vi "Create Screen.vi"(8 "error in (no error)":errorcluster caption="错误输入（无错误）", 11 "Screen 输入":refnum<class "Screen.lvclass"> caption="DNL_LabVIEW Object in") -> (0 "error out":errorcluster caption="错误输出", 3 "Screen 输出":refnum<class "Screen.lvclass"> caption="DNL_LabVIEW Object out")   [LabVIEW 2011, in "Screen.lvclass"]
uses:
  Screen.lvclass
  Screen.lvclass/Screen.ctl
  System.Windows.Forms
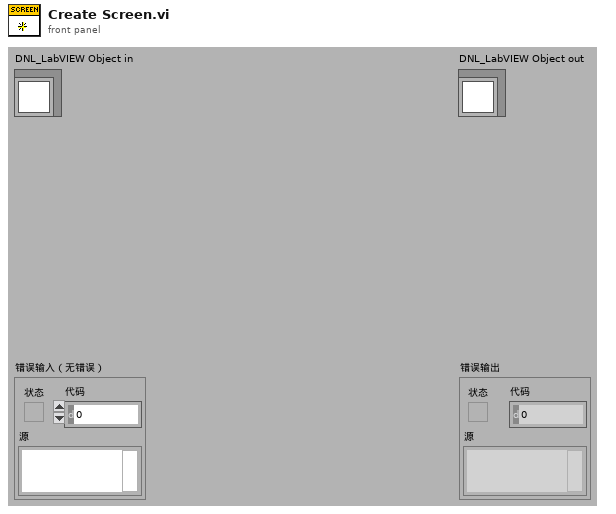
[diagram p1: front panel]
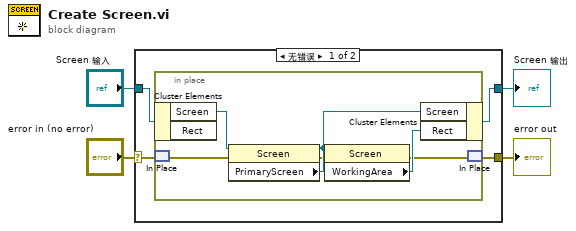
[diagram p0: block diagram]
diagram:
  n1 = case shown="无错误" "error in (no error)" {
    selector: "error in (no error)" -> [w7 w16]
    tunnel: [w6 w16] -> w3
    tunnel: [w5 w15] -> w1
    tunnel: "Screen 输入" -> [w8 w15]
    frame No Error {
      n2 = in-place {
        n3 = in-place-cluster #1(w8) -> ("Screen"=w14:refnum<k24>)  [unwired: 1 out]
        n4 = in-place-match #2(w7) -> (w13:errorcluster)
        n5 = property class="Screen"(reference=w14, error in=w13) -> (error out=w10:errorcluster, "PrimaryScreen"=w12:refnum<k24>)  [unwired: 1 out]
        n6 = property class="Screen"(reference=w12, error in=w10) -> (error out=w9:errorcluster, "WorkingArea"=w11:refnum<k24>)  [unwired: 1 out]
        n7 = in-place-cluster #1("Screen"=w12, "Rect"=w11) -> (w5:refnum<class "Screen.lvclass">)
        n8 = in-place-match #2(w9) -> (w6:errorcluster)
      }
    }
    frame Error {
    }
  }
  "error out" <- w3
  "Screen 输出" <- w1
